vi "GetStepAmplitudeNegative.vi"(8 "error in (no error)":errorcluster, 9 "Axis":i32, 10 "Output Refnum In":refnum<vi>, 11 "CmdLib In":refnum<k24>) -> (0 "error out":errorcluster, 1 "Step Amplitude":i32, 2 "GetStepAmplitudeNegative":bool, 3 "CmdLib Out":refnum<k24>)   [LabVIEW 2013]
uses:
  C:/Code/Apps/Utilities/AG-UC2-UC8/AG-UC2-UC8/Install/Samples/LabVIEW/LabVIEW 2013/CmdLibAgilis.dll
  CmdLibAgilis.dll
panel:
  in  "step amplitude":i32
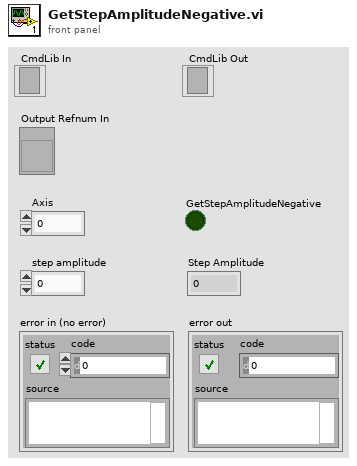
[diagram p1: front panel]
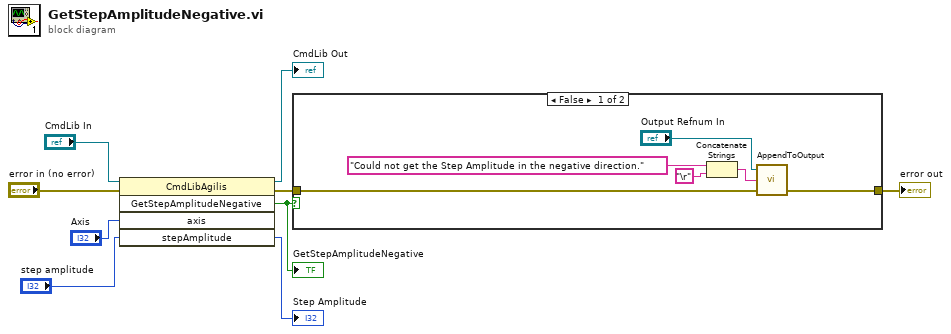
[diagram p0: block diagram]
diagram:
  n1 = invoke class="CmdLibAgilis" method="GetStepAmplitudeNegative"(reference="CmdLib In", error in="error in (no error)", "axis"="Axis", "stepAmplitude"="step amplitude") -> (reference out=→"CmdLib Out":refnum<k24>, error out=w2:errorcluster, "GetStepAmplitudeNegative"=w3:bool, "stepAmplitude"=→"Step Amplitude":i32)  [unwired: 1 in, 1 out]
  "GetStepAmplitudeNegative" <- w3
  n2 = case shown="False" w3 {
    tunnel: w2 -> [w13 w16]
    tunnel: [w12 w16] -> w1
    frame False {
      n3 = Concatenate Strings("Could not get the Step Amplitude in the negative direction.", "\r") -> (w11:string)
      n4 = call "AppendToOutput.vi"("error in"=w13, "Input String"=w11, "Output Refnum In"="Output Refnum In") -> ("error out"=w12:errorcluster)  [unwired: 1 in, 1 out]
    }
    frame True {
    }
  }
  "error out" <- w1
